vi "PH_GUI.set double GUI object.vi"(0 "Caption":string, 1 "visible (true)":bool=TRUE, 2 "GUI object Ref":refnum<vi>, 3 "value":dbl caption="Value", 4 "blinking (false)":bool, 5 "error in (no error)":errorcluster, 7 "Tip Strip [Empty]":string, 9 "Disabled (Enabled)":T1(ring)) -> (19 "error out":errorcluster)   [LabVIEW 2014, in "PH_Common.lvlib"]
doc: "Sets value and more for the referenced GUI object."
uses:
  PH_Common.lvlib
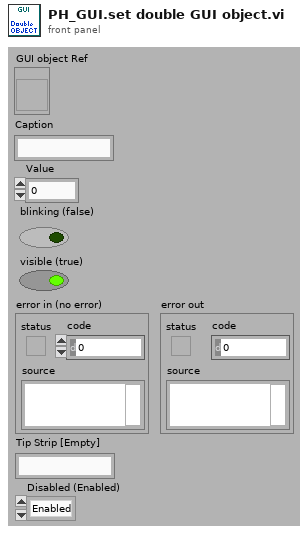
[diagram p1: front panel]
types:
  T1 = enum8{"Enabled", "Disabled", "Disabled and Grayed Out"}
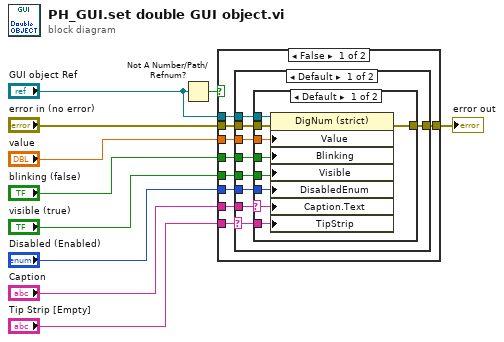
[diagram p0: block diagram]
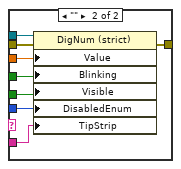
[diagram p2: hidden frame]
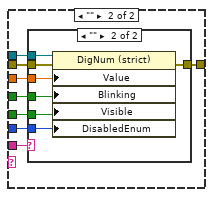
[diagram p3: hidden frame]
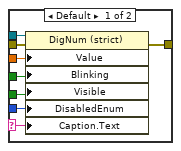
[diagram p4: hidden frame]
diagram:
  n1 = Not A Number/Path/Refnum?(number/path/refnum="GUI object Ref") -> (NaN/Path/Refnum?=w7:bool)
  n2 = case shown="False" w7 {
    tunnel: "GUI object Ref" -> [w18 _]
    tunnel: "error in (no error)" -> [w19 w69]
    tunnel: [w17 w69] -> w9
    tunnel: "value" -> [w16 _]
    tunnel: "blinking (false)" -> [w15 _]
    tunnel: "visible (true)" -> [w14 _]
    tunnel: "Caption" -> [w13 _]
    tunnel: "Disabled (Enabled)" -> [w12 _]
    tunnel: "Tip Strip [Empty]" -> [w11 _]
    frame False {
      n3 = case shown="Default" w11 {
        selector: w11 -> [w20 _]
        tunnel: w19 -> [w28 w53]
        tunnel: w18 -> [w27 w52]
        tunnel: [w26 w51] -> w17
        tunnel: w16 -> [w25 w50]
        tunnel: w15 -> [w24 w49]
        tunnel: w14 -> [w23 w48]
        tunnel: w13 -> [w22 w47]
        tunnel: w12 -> [w21 w46]
        frame Default {
          n4 = case shown="Default" w22 {
            selector: w22 -> [w31 _]
            tunnel: w28 -> [w37 w45]
            tunnel: w27 -> [w36 w44]
            tunnel: [w35 w43] -> w26
            tunnel: w25 -> [w34 w42]
            tunnel: w24 -> [w33 w41]
            tunnel: w23 -> [w32 w40]
            tunnel: w21 -> [w30 w39]
            tunnel: w20 -> [w29 w38]
            frame Default {
              n5 = property class="DigNum (strict)"(reference=w36, error in=w37, "Value"=w34, "Blinking"=w33, "Visible"=w32, "DisabledEnum"=w30, "Caption.Text"=w31, "TipStrip"=w29) -> (error out=w35:errorcluster)  [unwired: 1 out]
            }
            frame "" {
              n6 = property class="DigNum (strict)"(reference=w44, error in=w45, "Value"=w42, "Blinking"=w41, "Visible"=w40, "DisabledEnum"=w39, "TipStrip"=w38) -> (error out=w43:errorcluster)  [unwired: 1 out]
            }
          }
        }
        frame "" {
          n7 = case shown="\"\"" w47 {
            selector: w47 -> [w55 _]
            tunnel: w53 -> [w61 w68]
            tunnel: w52 -> [w60 w67]
            tunnel: [w59 w66] -> w51
            tunnel: w50 -> [w58 w65]
            tunnel: w49 -> [w57 w64]
            tunnel: w48 -> [w56 w63]
            tunnel: w46 -> [w54 w62]
            frame Default {
              n8 = property class="DigNum (strict)"(reference=w60, error in=w61, "Value"=w58, "Blinking"=w57, "Visible"=w56, "DisabledEnum"=w54, "Caption.Text"=w55) -> (error out=w59:errorcluster)  [unwired: 1 out]
            }
            frame "" {
              n9 = property class="DigNum (strict)"(reference=w67, error in=w68, "Value"=w65, "Blinking"=w64, "Visible"=w63, "DisabledEnum"=w62) -> (error out=w66:errorcluster)  [unwired: 1 out]
            }
          }
        }
      }
    }
    frame True {
    }
  }
  "error out" <- w9
